vi "Read Resource Name.vi"(8 "error in (no error)":errorcluster, 11 "CS++DeviceGUIActor in":refnum<class "CS++DeviceGUIActor.lvclass">) -> (0 "error out":errorcluster, 2 "Resource Name":string, 3 "CS++DeviceGUIActor out":refnum<class "CS++DeviceGUIActor.lvclass">)   [LabVIEW 2013, in "CS++DeviceGUIActor.lvlib" / "CS++DeviceGUIActor.lvclass"]
doc: "Specifies which instrument to use. \n\nFollowing info refers to VISA. Other instruments may have other naming conventions.\n\nInstruments that are powered on and connected to your computer are visible in the <B>VISA resource name</B> pull-down menu. Select the resource name from the <B>VISA resource name</B> pull-down menu. If your instrument does not appear in this list, enter the instrument descriptor using the following format: \n\nInterface Type[board index]::Address::INSTR. \n\n<B>Examples:</B>\n\n<B>GPIB:</B> GPIB::22::INSTR, GPIB board 0, primary address 22 \n\n<B>Serial:</B> COM1\n\n<B>TCP/IP Instr:</B> TCPIP::10.0.32.48::INSTR\n\n<B>TCP/IP Socket:</B> TCPIP::10.0.32.45::3800::SOCKET\n\n<B>USB Instr:</B> USB0::0x0957::0x0507::MY44000390::INSTR\n\n<B>USB Raw:</B> You must first link VISA to non-USBTMC instruments by using the VISA Driver Development Wizard\n\n<B>VISA Alias:</B> \"SampleInstr\" - Alias names are configured in MAX\n\nRefer to LabVIEW online help for more information on specifying a VISA resource name.\n\nThis value has been read at launch time of actor once."
uses:
  CS++DeviceGUIActor.lvclass
  CS++DeviceGUIActor.lvclass/CS++DeviceGUIActor.ctl
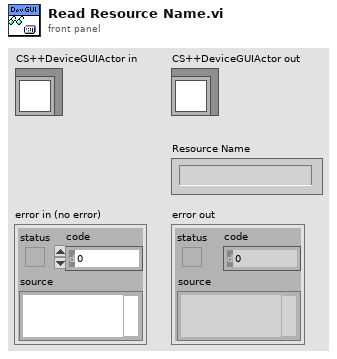
[diagram p1: front panel]
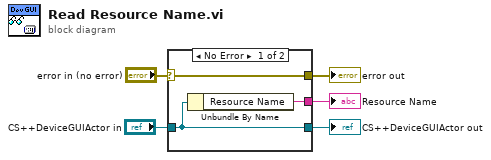
[diagram p0: block diagram]
diagram:
  n1 = case shown="No Error" "error in (no error)" {
    selector: "error in (no error)" -> [w8 w9]
    tunnel: [w8 w9] -> w4
    tunnel: [w7 w10] -> w2
    tunnel: "CS++DeviceGUIActor in" -> [w7 w10]
    tunnel: [w6 _] -> w1
    frame No Error {
      n2 = Unbundle By Name(w7) -> ("Resource Name"=w6:string)
    }
    frame Error {
    }
  }
  "error out" <- w4
  "CS++DeviceGUIActor out" <- w2
  "Resource Name" <- w1
